vi "getBackNode.vi"(8 "error in (no error)":errorcluster, 11 "LinkedList in":refnum<class "LinkedList.lvclass">) -> (0 "error out":errorcluster, 1 "ignore":bool, 2 "BackNode":refnum<data-value>, 3 "LinkedList out":refnum<class "LinkedList.lvclass">)   [LabVIEW 2013, in "LinkedList.lvclass"]
doc: "Retrieves the node at the back of the linked list."
uses:
  LinkedList.lvclass
  LLNode/LLNode.lvclass
  LinkedList.lvclass/LinkedList.ctl
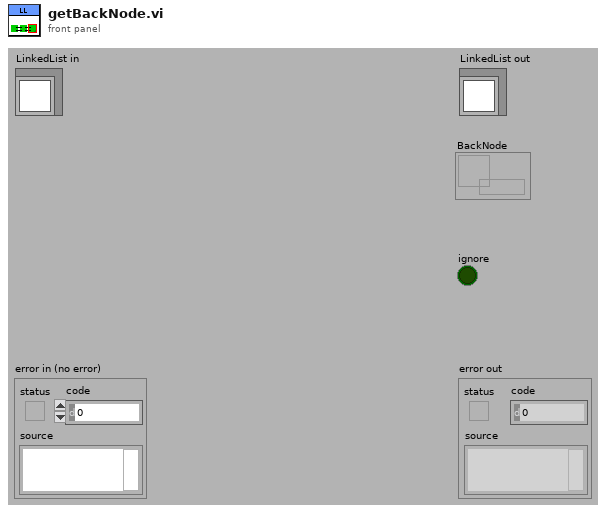
[diagram p1: front panel]
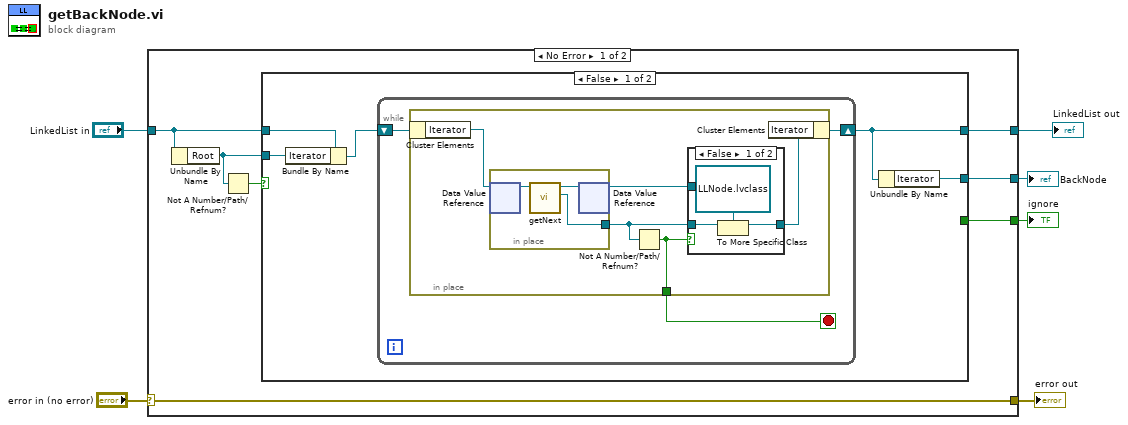
[diagram p0: block diagram]
diagram:
  n1 = case shown="No Error" "error in (no error)" {
    selector: "error in (no error)" -> [w13 w37]
    tunnel: [w13 w37] -> w3
    tunnel: [w9 w36] -> w4
    tunnel: "LinkedList in" -> [w12 w36]
    tunnel: [w8 _] -> w2
    tunnel: [w7 _] -> w1
    frame No Error {
      n2 = Unbundle By Name(w12) -> ("Root"=w10:refnum<data-value>)
      n3 = Not A Number/Path/Refnum?(number/path/refnum=w10) -> (NaN/Path/Refnum?=w11:bool)
      n4 = case shown="False" w11 {
        selector: w11 -> [_ w34]
        tunnel: w10 -> [w18 _]
        tunnel: w12 -> [w17 w35]
        tunnel: [w14 w35] -> w9
        tunnel: [w15 _] -> w8
        tunnel: [_ w34] -> w7
        frame False {
          n5 = Bundle By Name(cluster=w17, "Iterator"=w18) -> (w16:refnum<class "LinkedList.lvclass">)
          n6 = while {
            shift-right: [w20] -> w14
            shift-left: w16 -> [w21]
            stop <- w19 stop-if-true
            n7 = in-place {
              in-place-border: [w23] -> w19
              n8 = in-place-cluster #1(w21) -> ("Iterator"=w26:refnum<data-value>)
              n9 = in-place {
                in-place-border: [w31] -> w25
                n10 = in-place-dvr #2(w26) -> (w33:refnum<class "LLNode.lvclass">)  [unwired: 1 out]
                n11 = call "getNext.vi"("LLNode in"=w33) -> ("next"=w31:refnum<data-value>, "LLNode out"=w32:refnum<class "LLNode.lvclass">)  [unwired: 8 in, 1 out]
                n12 = in-place-dvr #2(w32) -> (w22:refnum<data-value>)  [unwired: 1 out]
              }
              n13 = Not A Number/Path/Refnum?(number/path/refnum=w25) -> (NaN/Path/Refnum?=w23:bool)
              n14 = case shown="False" w23 {
                tunnel: w25 -> [w29 _]
                tunnel: [w27 w30] -> w24
                tunnel: w22 -> [_ w30]
                frame False {
                  n15 = To More Specific Class(target class=refnum<data-value> refnum ("Root"), reference=w29) -> (specific class reference=w27:refnum<data-value>)  [unwired: 1 in, 1 out]
                }
                frame True {
                }
              }
              n16 = in-place-cluster #1("Iterator"=w24) -> (w20:refnum<class "LinkedList.lvclass">)
            }
          }
          n17 = Unbundle By Name(w14) -> ("Iterator"=w15:refnum<data-value>)
        }
        frame True {
        }
      }
    }
    frame Error {
    }
  }
  "error out" <- w3
  "LinkedList out" <- w4
  "BackNode" <- w2
  "ignore" <- w1
